vi "Autonomous_Load.vi"(0 "Number of Commands":i32, 5 "Subsystems":string[](array[string]), 7 "Commands":string[](array[string]), 9 "Inputs":string[][](array[string]), 11 "error in":errorcluster) -> (4 "Queue_Key":refnum<queue>, 6 "Autonomous_Queue":refnum<queue>, 15 "errror out":errorcluster)   [LabVIEW 2019]
uses:
  Autonomous Utilities/Queue_Key_Data.ctl
  RobotSubsystemsCluster.ctl
  Subsystems/Drive/DriveExecuteCluster.ctl
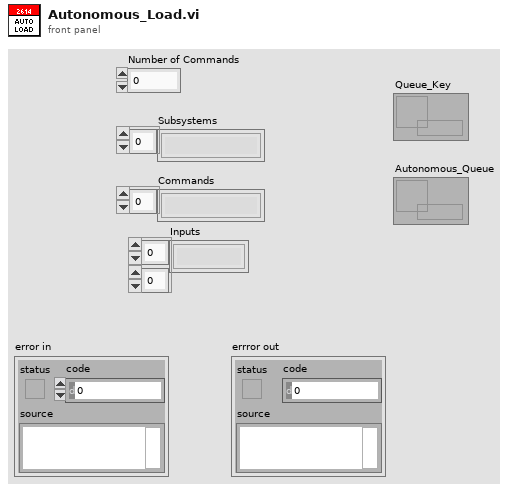
[diagram p1: front panel]
types:
  T1 = typedef "RobotSubsystemsCluster.ctl" = cluster{"Drive Execute Cluster":T2}
  T2 = typedef "DriveExecuteCluster.ctl" = cluster{"Front/Back":dbl, "Turn":dbl, "Drive_Control_Type":enum16{"PercentVoltage", "SpeedControl", "Command_Distance"}, "Step":dbl, "Parameter_1":dbl, "Parameter_2":dbl, "Parameter_3":dbl, "Parameter_4":dbl, "Auto_Notifier":refnum<notifier>}
  T3 = typedef "Queue_Key_Data.ctl" = cluster{"Operation Notifier":refnum<notifier>, "Subsystem":string, "Concurrent":bool}
  T4 = enum16{"PercentVoltage", "SpeedControl", "Command_Distance"}
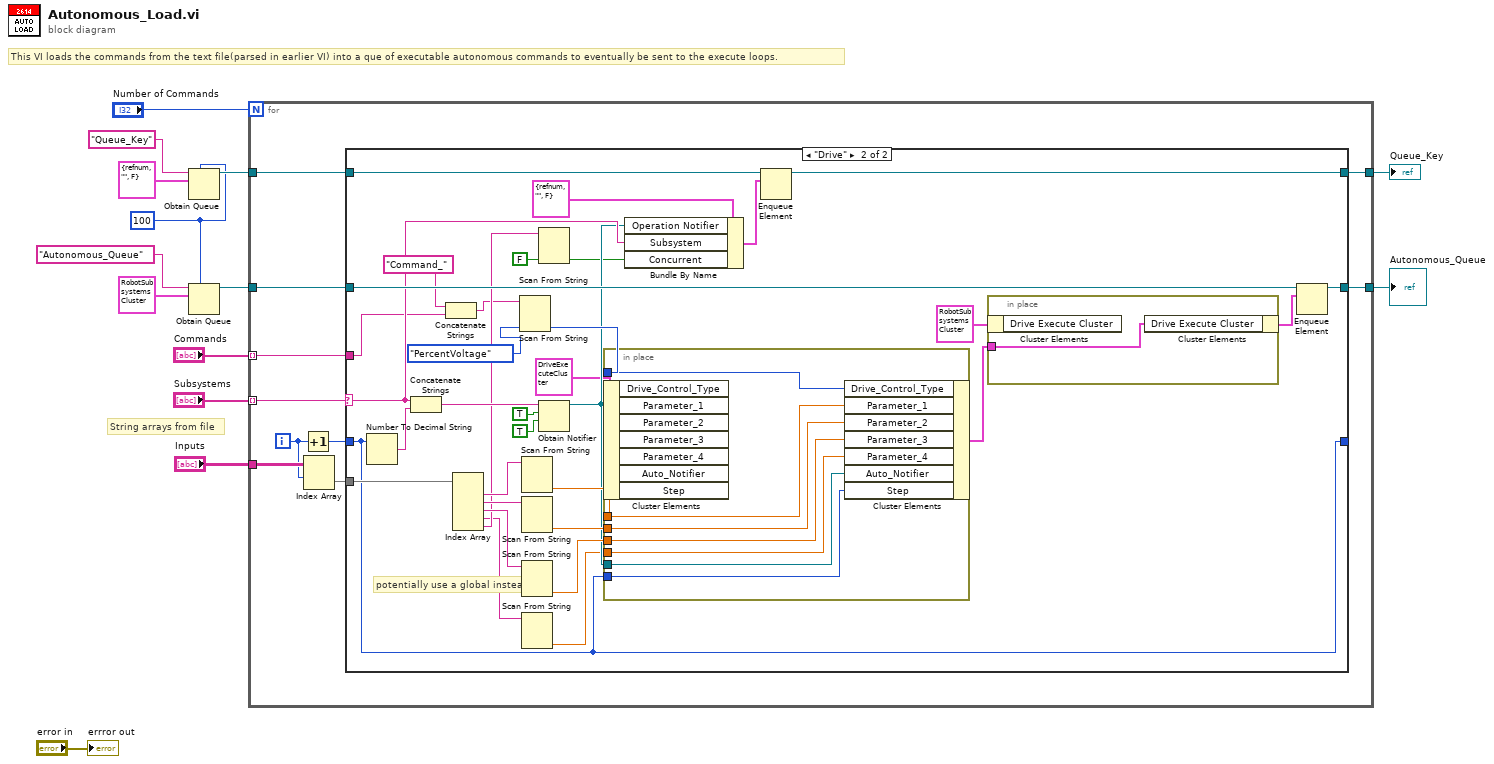
[diagram p0: block diagram]
diagram:
  w6 = 100 ("max queue size (-1, unlimited)")
  # "This VI loads the commands from the text file(parsed in earlier VI) into a que of executable autonomous commands to eventually be sent to the execute loops."
  # "String arrays from file"
  n1 = Obtain Queue(max queue size (-1, unlimited)=w6, name (unnamed)="Queue_Key", element data type=T3 {"Operation Notifier"=refnum, "Subsystem"="", "Concurrent"=FALSE} ("Queue Key Data")) -> (queue out=w12:refnum<queue>)  [unwired: 2 in, 2 out]
  n2 = Obtain Queue(max queue size (-1, unlimited)=w6, name (unnamed)="Autonomous_Queue", element data type=T1 {"Drive Execute Cluster"={"Front/Back"=0.0, "Turn"=0.0, "Drive_Control_Type"=enum."PercentVoltage", "Step"=0.0, "Parameter_1"=0.0, "Parameter_2"=0.0, "Parameter_3"=0.0, "Parameter_4"=0.0, "Auto_Notifier"=refnum}}) -> (queue out=w7:refnum<queue>)  [unwired: 2 in, 2 out]
  n3 = for {
    N: "Number of Commands" -> [_]
    tunnel: w12 -> [w24]
    tunnel: "Subsystems" -> [w23] mode=indexing
    tunnel: "Commands" -> [w22] mode=indexing
    tunnel: "Inputs" -> [w18]
    tunnel: [w21] -> w4
    tunnel: w7 -> [w20]
    tunnel: [w15] -> w1
    i -> [w16]
    n4 = Increment(x=w16) -> (x+1=w19:i32)
    n5 = Index Array(array=w18, index (row)=w16) -> (element=w17:string[])  [unwired: 1 in]
    n6 = case shown="\"Drive\"" w23 {
      selector: w23 -> [_ w41]
      tunnel: w24 -> [w26 w44]
      tunnel: w22 -> [_ w30]
      tunnel: [w27 w45] -> w15
      tunnel: [w26 w37] -> w21
      tunnel: w20 -> [w27 w48]
      tunnel: w19 -> [w25 w55]
      tunnel: [w25 w55] -> _
      tunnel: w17 -> [_ w56]
      frame "No Op", Default {
      }
      frame "Drive" {
        # "potentially use a global instead"
        n7 = Number To Decimal String(number=w55) -> (decimal integer string=w59:string)  [unwired: 1 in]
        n8 = Concatenate Strings(w41, w59) -> (w58:string)
        n9 = Concatenate Strings("Command_" ("string"), w30) -> (w31:string)
        n10 = Index Array(array=w56) -> (element #1=w54:string, element #2=w52:string, element #3=w49:string, element #4=w35:string, element #5=w36:string)  [unwired: 5 in]
        n11 = Scan From String(input string=w31, default 1=T4."PercentVoltage" ("Drive_Control_Type")) -> (output 1=w57:T4)  [unwired: 3 in, 3 out]
        n12 = Scan From String(input string=w54) -> (output 1=w53:dbl)  [unwired: 4 in, 3 out]
        n13 = Scan From String(input string=w52) -> (output 1=w51:dbl)  [unwired: 4 in, 3 out]
        n14 = Scan From String(input string=w49) -> (output 1=w50:dbl)  [unwired: 4 in, 3 out]
        n15 = Scan From String(input string=w35) -> (output 1=w34:dbl)  [unwired: 4 in, 3 out]
        n16 = Scan From String(input string=w36, default 1=FALSE) -> (output 1=w38:bool)  [unwired: 3 in, 3 out]
        n17 = Obtain Notifier(name (unnamed)=w58, notification data type=TRUE ("create if not found? (T)"), create if not found? (T)=TRUE) -> (notifier out=w40:refnum<notifier>)  [unwired: 1 in, 2 out]
        n18 = in-place {
          in-place-border: w57 -> [w69]
          in-place-border: w40 -> [w68]
          in-place-border: w55 -> [w67]
          in-place-border: w53 -> [w66]
          in-place-border: w51 -> [w65]
          in-place-border: w50 -> [w64]
          in-place-border: w34 -> [w63]
          n19 = in-place-cluster #1(T2 {"Front/Back"=0.0, "Turn"=0.0, "Drive_Control_Type"=enum."PercentVoltage", "Step"=0.0, "Parameter_1"=0.0, "Parameter_2"=0.0, "Parameter_3"=0.0, "Parameter_4"=0.0, "Auto_Notifier"=refnum} ("Drive Execute Cluster")) -> ()  [unwired: 7 out]
          n20 = in-place-cluster #1("Drive_Control_Type"=w69, "Parameter_1"=w66, "Parameter_2"=w65, "Parameter_3"=w64, "Parameter_4"=w63, "Auto_Notifier"=w68, "Step"=w67) -> (w47:T2)
        }
        n21 = Bundle By Name(cluster=T3 {"Operation Notifier"=refnum, "Subsystem"="", "Concurrent"=FALSE} ("Queue Key Data"), "Operation Notifier"=w40, "Subsystem"=w41, "Concurrent"=w38) -> (w43:T3)
        n22 = Enqueue Element(queue=w44, element=w43) -> (queue out=w37:refnum<queue>)  [unwired: 2 in, 2 out]
        n23 = in-place {
          in-place-border: w47 -> [w62]
          n24 = in-place-cluster #2(T1 {"Drive Execute Cluster"={"Front/Back"=0.0, "Turn"=0.0, "Drive_Control_Type"=enum."PercentVoltage", "Step"=0.0, "Parameter_1"=0.0, "Parameter_2"=0.0, "Parameter_3"=0.0, "Parameter_4"=0.0, "Auto_Notifier"=refnum}}) -> ()  [unwired: 1 out]
          n25 = in-place-cluster #2("Drive Execute Cluster"=w62) -> (w46:T1)
        }
        n26 = Enqueue Element(queue=w48, element=w46) -> (queue out=w45:refnum<queue>)  [unwired: 2 in, 2 out]
      }
    }
  }
  "Queue_Key" <- w4
  "Autonomous_Queue" <- w1
  "errror out" <- "error in"
